vi "DeltaRCMotorControl.vi"(8 "error in (no error)":errorcluster, 9 "Theta3":dbl, 10 "Theta2":dbl, 11 "Theta1":dbl) -> (0 "error out":errorcluster)   [LabVIEW 2019]
uses:
  KNRm_ReMi_OS6_436Motor.lvlibp/KNRm_ReMi_Toolkit/IO/LowLevel/IO_Channel_RC.ctl
  math/Global 1.vi
  KNRm_ReMi_OS6_436Motor.lvlibp
panel:
  out "coerced(x)":dbl
  out "x/y":dbl
  out "x+y":dbl
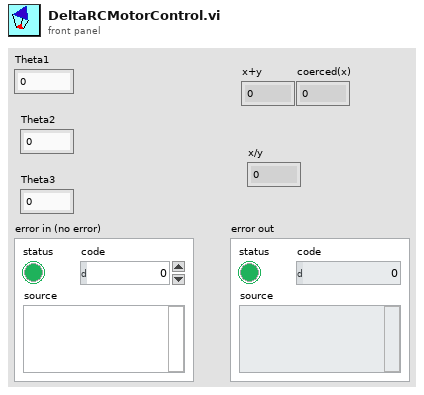
[diagram p1: front panel]
types:
  T1 = typedef "KNRm_ReMi_OS6_436Motor.lvlibp/IO_Channel_RC.ctl" = enum16{"RC1", "RC2", "S1(EXTIOB)", "S2(EXTIOB)", "S3(EXTIOB)", "S4(EXTIOB)", "S5(EXTIOB)", "S6(EXTIOB)"}
  T2 = cluster{"等比調整到角度正確":cluster{"S1":dbl, "S2":dbl, "S3":dbl, "S4":dbl, "S5":dbl}, "補償角度到0度是水平":cluster{"S1":dbl, "S2":dbl, "S3":dbl, "S4":dbl, "S5":dbl}}
  T3 = cluster{"S1":dbl, "S2":dbl, "S3":dbl, "S4":dbl, "S5":dbl}
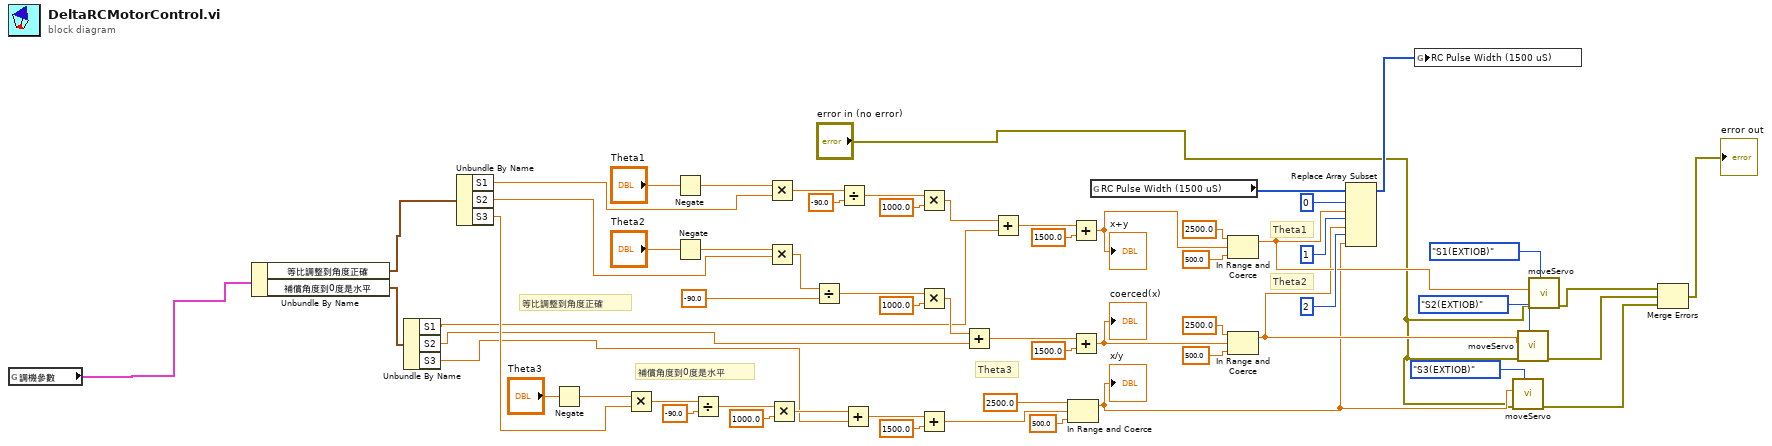
[diagram p0: block diagram]
diagram:
  # "補償角度到0度是水平"
  # "等比調整到角度正確"
  # "Theta2"
  # "Theta3"
  # "Theta1"
  n1 = global read "Global 1.vi" "調機參數"() -> (w1:T2)
  n2 = Unbundle By Name(w1) -> ("等比調整到角度正確"=w9:T3, "補償角度到0度是水平"=w8:T3)
  n3 = Unbundle By Name(w8) -> ("S1"=w4:dbl, "S2"=w3:dbl, "S3"=w2:dbl)
  n4 = Unbundle By Name(w9) -> ("S1"=w7:dbl, "S2"=w6:dbl, "S3"=w5:dbl)
  n5 = Negate(x="Theta3") -> (-x=w35:dbl)
  n6 = Multiply(x=w35, y=w5) -> (x*y=w33:dbl)
  n7 = Negate(x="Theta1") -> (-x=w36:dbl)
  n8 = Negate(x="Theta2") -> (-x=w37:dbl)
  n9 = Divide(x=w33, y=-90.0) -> (x/y=w58:dbl)
  n10 = Multiply(x=w36, y=w7) -> (x*y=w34:dbl)
  n11 = Multiply(x=w37, y=w6) -> (x*y=w32:dbl)
  n12 = Multiply(x=w58, y=1000.0) -> (x*y=w27:dbl)
  n13 = Divide(x=w32, y=-90.0) -> (x/y=w50:dbl)
  n14 = Divide(x=w34, y=-90.0) -> (x/y=w54:dbl)
  n15 = Add(x=w27, y=w2) -> (x+y=w26:dbl)
  n16 = Multiply(x=w54, y=1000.0) -> (x*y=w29:dbl)
  n17 = Multiply(x=w50, y=1000.0) -> (x*y=w31:dbl)
  n18 = Add(x=w26, y=1500.0) -> (x+y=w43:dbl)
  n19 = Add(x=w31, y=w3) -> (x+y=w30:dbl)
  n20 = Add(x=w29, y=w4) -> (x+y=w28:dbl)
  n21 = In Range and Coerce(upper limit=2500.0, x=w43, lower limit=500.0) -> (coerced(x)=w11:dbl)  [unwired: 1 out]
  "x/y" <- w11
  n22 = Add(x=w28, y=1500.0) -> (x+y=w42:dbl)
  "x+y" <- w42
  n23 = Add(x=w30, y=1500.0) -> (x+y=w41:dbl)
  "coerced(x)" <- w41
  n24 = global read "Global 1.vi" "RC Pulse Width (1500 uS)"() -> (w25:u16[])
  n25 = In Range and Coerce(upper limit=2500.0, x=w42, lower limit=500.0) -> (coerced(x)=w13:dbl)  [unwired: 1 out]
  n26 = In Range and Coerce(upper limit=2500.0, x=w41, lower limit=500.0) -> (coerced(x)=w12:dbl)  [unwired: 1 out]
  n27 = Replace Array Subset(array=w25, new element #1=w13, index #1=0 ("index"), new element #2=w12, index #2=1 ("index"), new element #3=w11, index #3=2 ("index")) -> (w23:u16[])
  n28 = global write "Global 1.vi" "RC Pulse Width (1500 uS)"(w23) -> ()
  n29 = call "moveServo.vi"("Channel"=IO_Channel_RC."S3(EXTIOB)", "error in (no error)"="error in (no error)", "Servo Position (us)"=w11) -> ("error out"=w15:errorcluster)  [unwired: 8 in]
  n30 = call "moveServo.vi"("Channel"=IO_Channel_RC."S2(EXTIOB)", "error in (no error)"="error in (no error)", "Servo Position (us)"=w12) -> ("error out"=w16:errorcluster)  [unwired: 8 in]
  n31 = call "moveServo.vi"("Channel"=IO_Channel_RC."S1(EXTIOB)", "error in (no error)"="error in (no error)", "Servo Position (us)"=w13) -> ("error out"=w17:errorcluster)  [unwired: 8 in]
  n32 = Merge Errors(w17, w16, w15) -> (→"error out":errorcluster)
